vi "运维调试_采配水.vi"() -> ()   [LabVIEW 2016, in "PLC.lvlib"]
uses:
  PLC.lvlib
  <vilib>/Plasmionique/MB Master/MB_Master/MB_Master.lvclass
  <vilib>/Utility/miscctls.llb/LVPointTypeDef.ctl
  <vilib>/Plasmionique/MB Master/MB_Master_Serial/MB_Master_Serial.lvclass
  C:/Program Files (x86)/National Instruments/LabVIEW 2016/vi.lib/Plasmionique/MB Master/MB_Master/MB_Master.lvclass
  <vilib>/Instr/_visa.llb/VISA Configure Serial Port (Instr).vi
  <vilib>/NI/Modbus Library/API/Wrapper/Create TCP Slave.vi
  <vilib>/NI/Modbus Library/API/Slave/Modbus Slave.lvclass
  <vilib>/Plasmionique/MB Master/MB Master.lvlib
  <vilib>/NI/Modbus Library/API/Wrapper/API Main.lvlib
panel:
  out "Registers":u16[](array[numeric])
  out "R118":i16 caption="多参数沉淀时间"
  in  "看门狗启用":bool
  out "R117":i16 caption="看门狗设置值"
  out "R33":i16 caption="看门狗计时器"
  in  "下载模式":bool
  in  "R116":i16(ring) caption="储水水体选择" items=["自来水", "采水泵"]
  out "当前启动泵号":u16(ring) items=["1号水样泵", "2号水样泵"]
  out "R113":i16 caption="储水时间设定"
  out "R25":i16
  in  "V14NC":bool
  out "R24":i16
  in  "V14NO":bool
  out "X2":bool caption="X1"
  out "采配水版本号":string
  out "R23":i16 caption="清洗频次计数"
  out "R112":i16 caption="清洗频次设定"
  out "R22":i16
  in  "V13NC":bool
  out "R111":i16 caption="排液时间"
  out "通讯故障":bool
  out "R21":i16
  in  "V13NO":bool
  out "R20":i16
  in  "M1-2":bool
  in  "潜水泵工作模式":u16(ring) items=["泵1单泵单管路", "泵2单泵单管路", "潜水泵双泵双管路", "自吸泵双泵双管路"]
  out "X11":bool caption="废液报警"
  out "X10":bool caption="自来水检测"
  out "X9":bool caption="泵2过载报警"
  out "X8":bool caption="泵1过载报警"
  out "X7":bool caption="断电检测"
  out "X6":bool caption="开门检测"
  out "X5":bool caption="烟雾检测"
  out "X4":bool caption="漏水检测"
  out "X3":bool caption="进样检测"
  out "X1":bool
  out "X0":bool caption="采样池液位开关"
  out "R109":i16 caption="配水时间"
  out "集成报警信息":string
  out "R108":i16 caption="自来水报警"
  out "R107":i16 caption="采水池液位报警设置"
  out "R106":i16 caption="进样超时设置"
  out "R105":i16 caption="二级清洗时间"
  out "R104":i16 caption="一级清洗时间"
  out "R103":i16 caption="外部管路清洗时间"
  out "R102":i16 caption="静置沉淀时间"
  out "R101":i16 caption="内部管路润洗时间"
  out "R100":i16 caption="外部管路润洗时间"
  out "R2":i16
  out "R1":i16
  out "多列列表框":i32(listbox)
  out "R19":i16
  in  "V6":bool
  out "R18":i16
  in  "V5":bool
  out "R17":i16
  in  "V4":bool
  out "R16":i16
  in  "V3":bool
  out "R15":i16
  in  "V2":bool
  out "R14":i16
  in  "M2":bool
  out "R13":i16
  in  "V1":bool
  out "R12":i16
  in  "M1-1":bool
  in  "返回":bool
  in  "参数设置":bool
  in  "单步启动":bool
  in  "启动":bool
  in  "停止":bool
  # "看门狗设置"
  # "S"
  # "S"
  # "S"
  # "S"
  # "次"
  # "次"
  # "S"
  # "S"
  # "S"
  # "S"
  # "S"
  # "S"
  # "S"
  # "S"
  # "S"
  # "S"
  # "S"
  # "单步计时："
  # "s"
  # "流程计时："
  # "s"
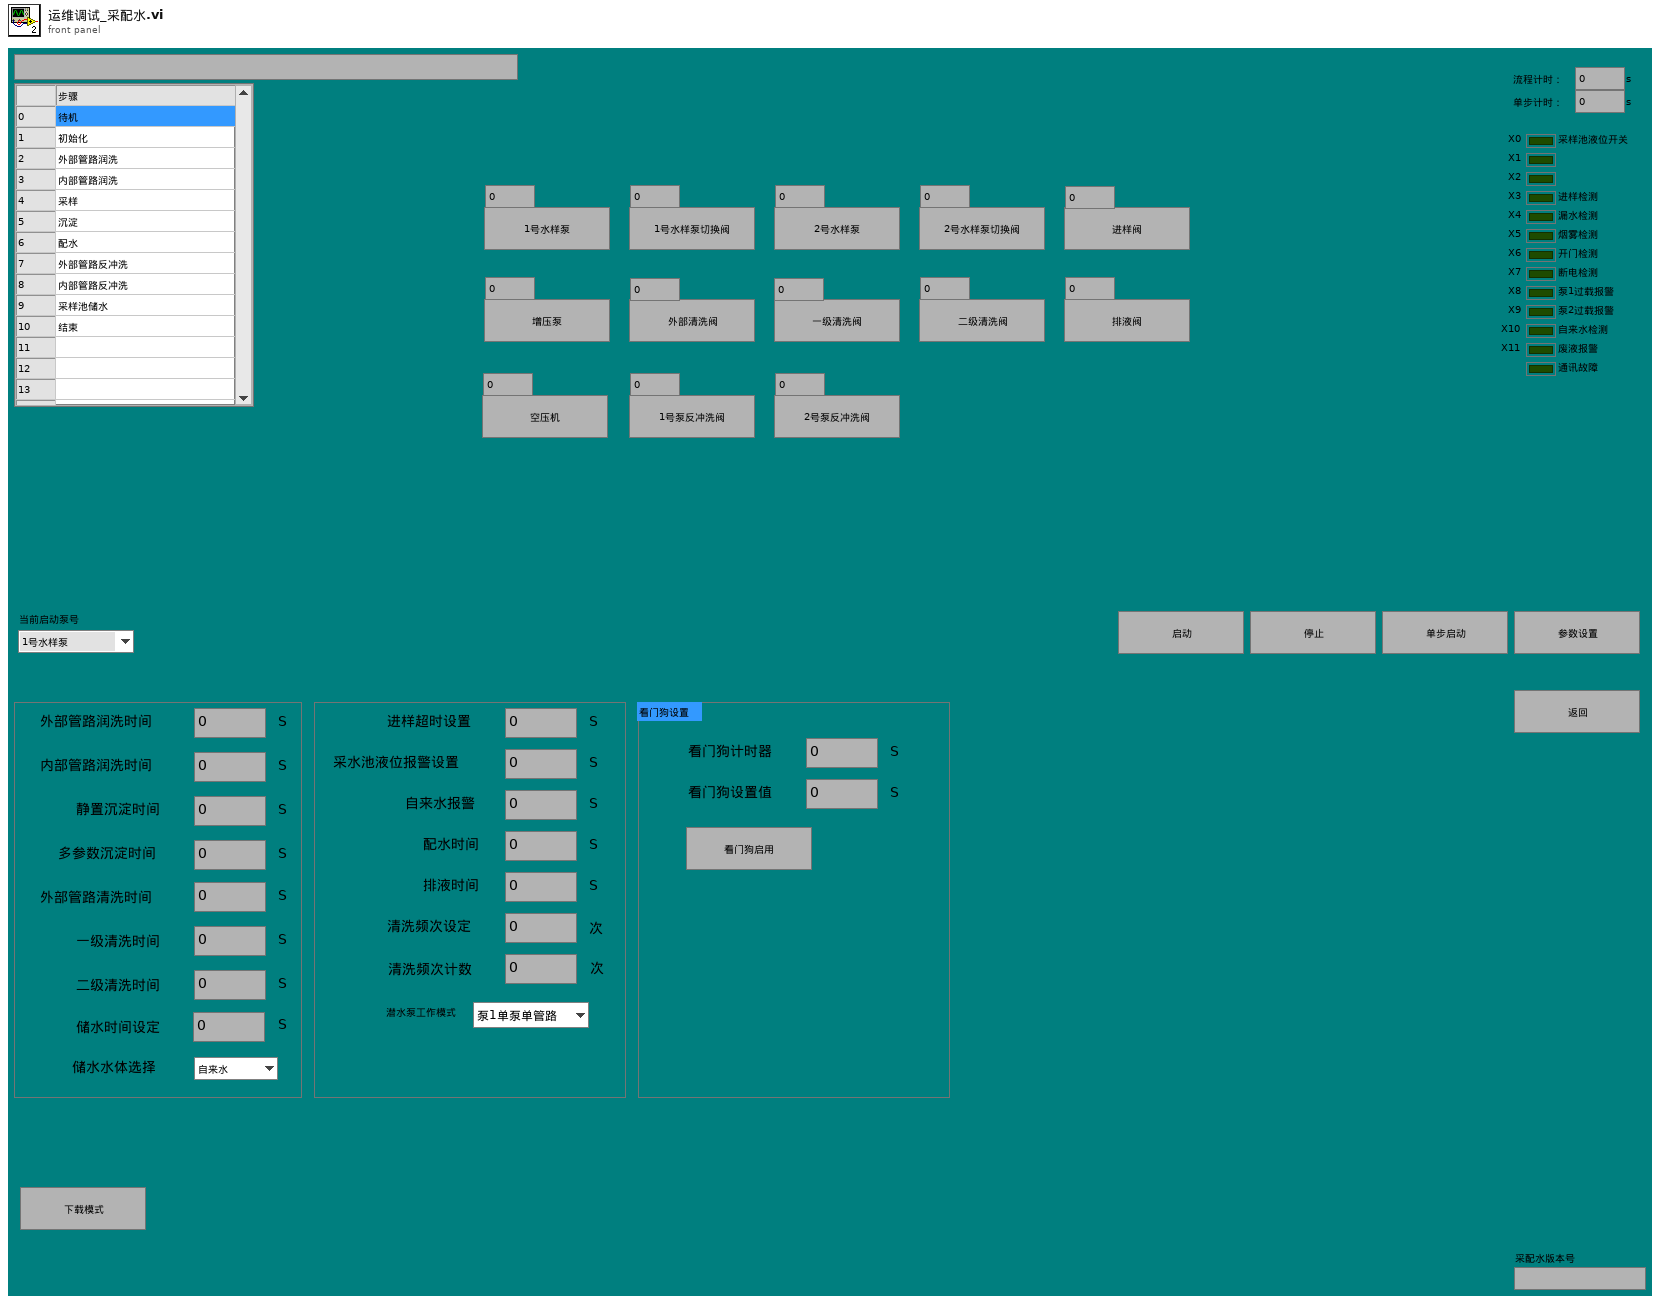
[diagram p1: front panel]
types:
  T1 = typedef "LVPointTypeDef.ctl" = cluster{"Horizontal":i16, "Vertical":i16}
  T2 = cluster{"命令":string, "数据":cluster{"starting address":u16, "holding register value":u16}}
  T3 = cluster{"时间标识":timestamp, "设备":string, "日志信息":string}
  T4 = cluster{"R0":i16, "R1":i16, "R2":i16, "R3":i16, "R4":i16, "R5":i16, "R6":i16, "R7":i16, "R8":i16, "R9":i16, "R10":i16, "R11":i16, "R12":i16, "R13":i16, "R14":i16, "R15":i16, "R16":i16, "R17":i16, "R18":i16, "R19":i16, "R20":i16, "R21":i16, "R22":i16, "R23":i16, "R24":i16, "R25":i16, "R26":i16, "R27":i16, "R28":i16, "R29":i16, "R30":i16, "R31":i16, "R32":i16, "R33":i16, "R34":i16}
  T5 = cluster{"R100":i16, "R101":i16, "R102":i16, "R103":i16, "R104":i16, "R105":i16, "R106":i16, "R107":i16, "R108":i16, "R109":i16, "R110":i16, "R111":i16, "R112":i16, "R113":i16, "R114":i16, "R115":i16, "R116":i16, "R117":i16, "R118":i16, "R119":i16}
  T6 = cluster{"seconds since 1Jan1904":timestamp, "table输入":string, string, "table输入":string}
  T7 = cluster{"时间标识":timestamp, "设备":string, "日志信息":string, "流程参数":string}
  T8 = cluster{"命令":string, cluster{"starting address":u16, "holding register value":u16}}
  T9 = cluster{"命令":string, "数据":cluster{"starting address":u16, "holding register values":u16[]}}
  T10 = cluster{"命令":string, "data":cluster{"starting address":u16, "coil values":bool[]}}
  T11 = cluster{"测试模式":enum16{"正常测试", "集成干预"}, "参数启用":cluster{"氨氮":bool, "总磷总氮":bool, "CODMn":bool, "CODcr":bool, "多参数":bool, "超标留样":bool}}
  T12 = enum32{"Bad", "Idle", "Run top level", "Running"}
  T13 = cluster{"baud rate (bps)":u32, "stop bits":u16, "parity":u16, "flow control":u16, "timeout":u32, "retries":i32}
  T14 = cluster{"starting address":u16, "holding register values":u16[]}
  T15 = cluster{"starting address":u16, "holding register value":u16}
  T16 = cluster{"starting address":u16, "coil values":bool[]}
  T17 = cluster{"Registers[0]":u16, "Registers[1]":u16, "Registers[2]":u16, "Registers[3]":u16, "Registers[4]":u16, "Registers[5]":u16, "Registers[6]":u16, "Registers[7]":u16, "Registers[8]":u16, "Registers[9]":u16, "Registers[10]":u16, "Registers[11]":u16, "Registers[12]":u16, "Registers[13]":u16, "Registers[14]":u16, "Registers[15]":u16, "Registers[16]":u16, "Registers[17]":u16, "Registers[18]":u16, "Registers[19]":u16, "Registers[20]":u16, "Registers[21]":u16, "Registers[22]":u16, "Registers[23]":u16, "Registers[24]":u16, "Registers[25]":u16, "Registers[26]":u16, "Registers[27]":u16, "Registers[28]":u16, "Registers[29]":u16, "Registers[30]":u16, "Registers[31]":u16, "Registers[32]":u16, "Registers[33]":u16, "Registers[34]":u16}
  T18 = cluster{"Registers[0]":u16, "Registers[1]":u16, "Registers[2]":u16, "Registers[3]":u16, "Registers[4]":u16, "Registers[5]":u16}
  T19 = cluster{"Registers[0]":u16, "Registers[1]":u16, "Registers[2]":u16, "Registers[3]":u16, "Registers[4]":u16, "Registers[5]":u16, "Registers[6]":u16, "Registers[7]":u16, "Registers[8]":u16, "Registers[9]":u16, "Registers[10]":u16, "Registers[11]":u16, "Registers[12]":u16, "Registers[13]":u16, "Registers[14]":u16, "Registers[15]":u16, "Registers[16]":u16, "Registers[17]":u16, "Registers[18]":u16, "Registers[19]":u16}
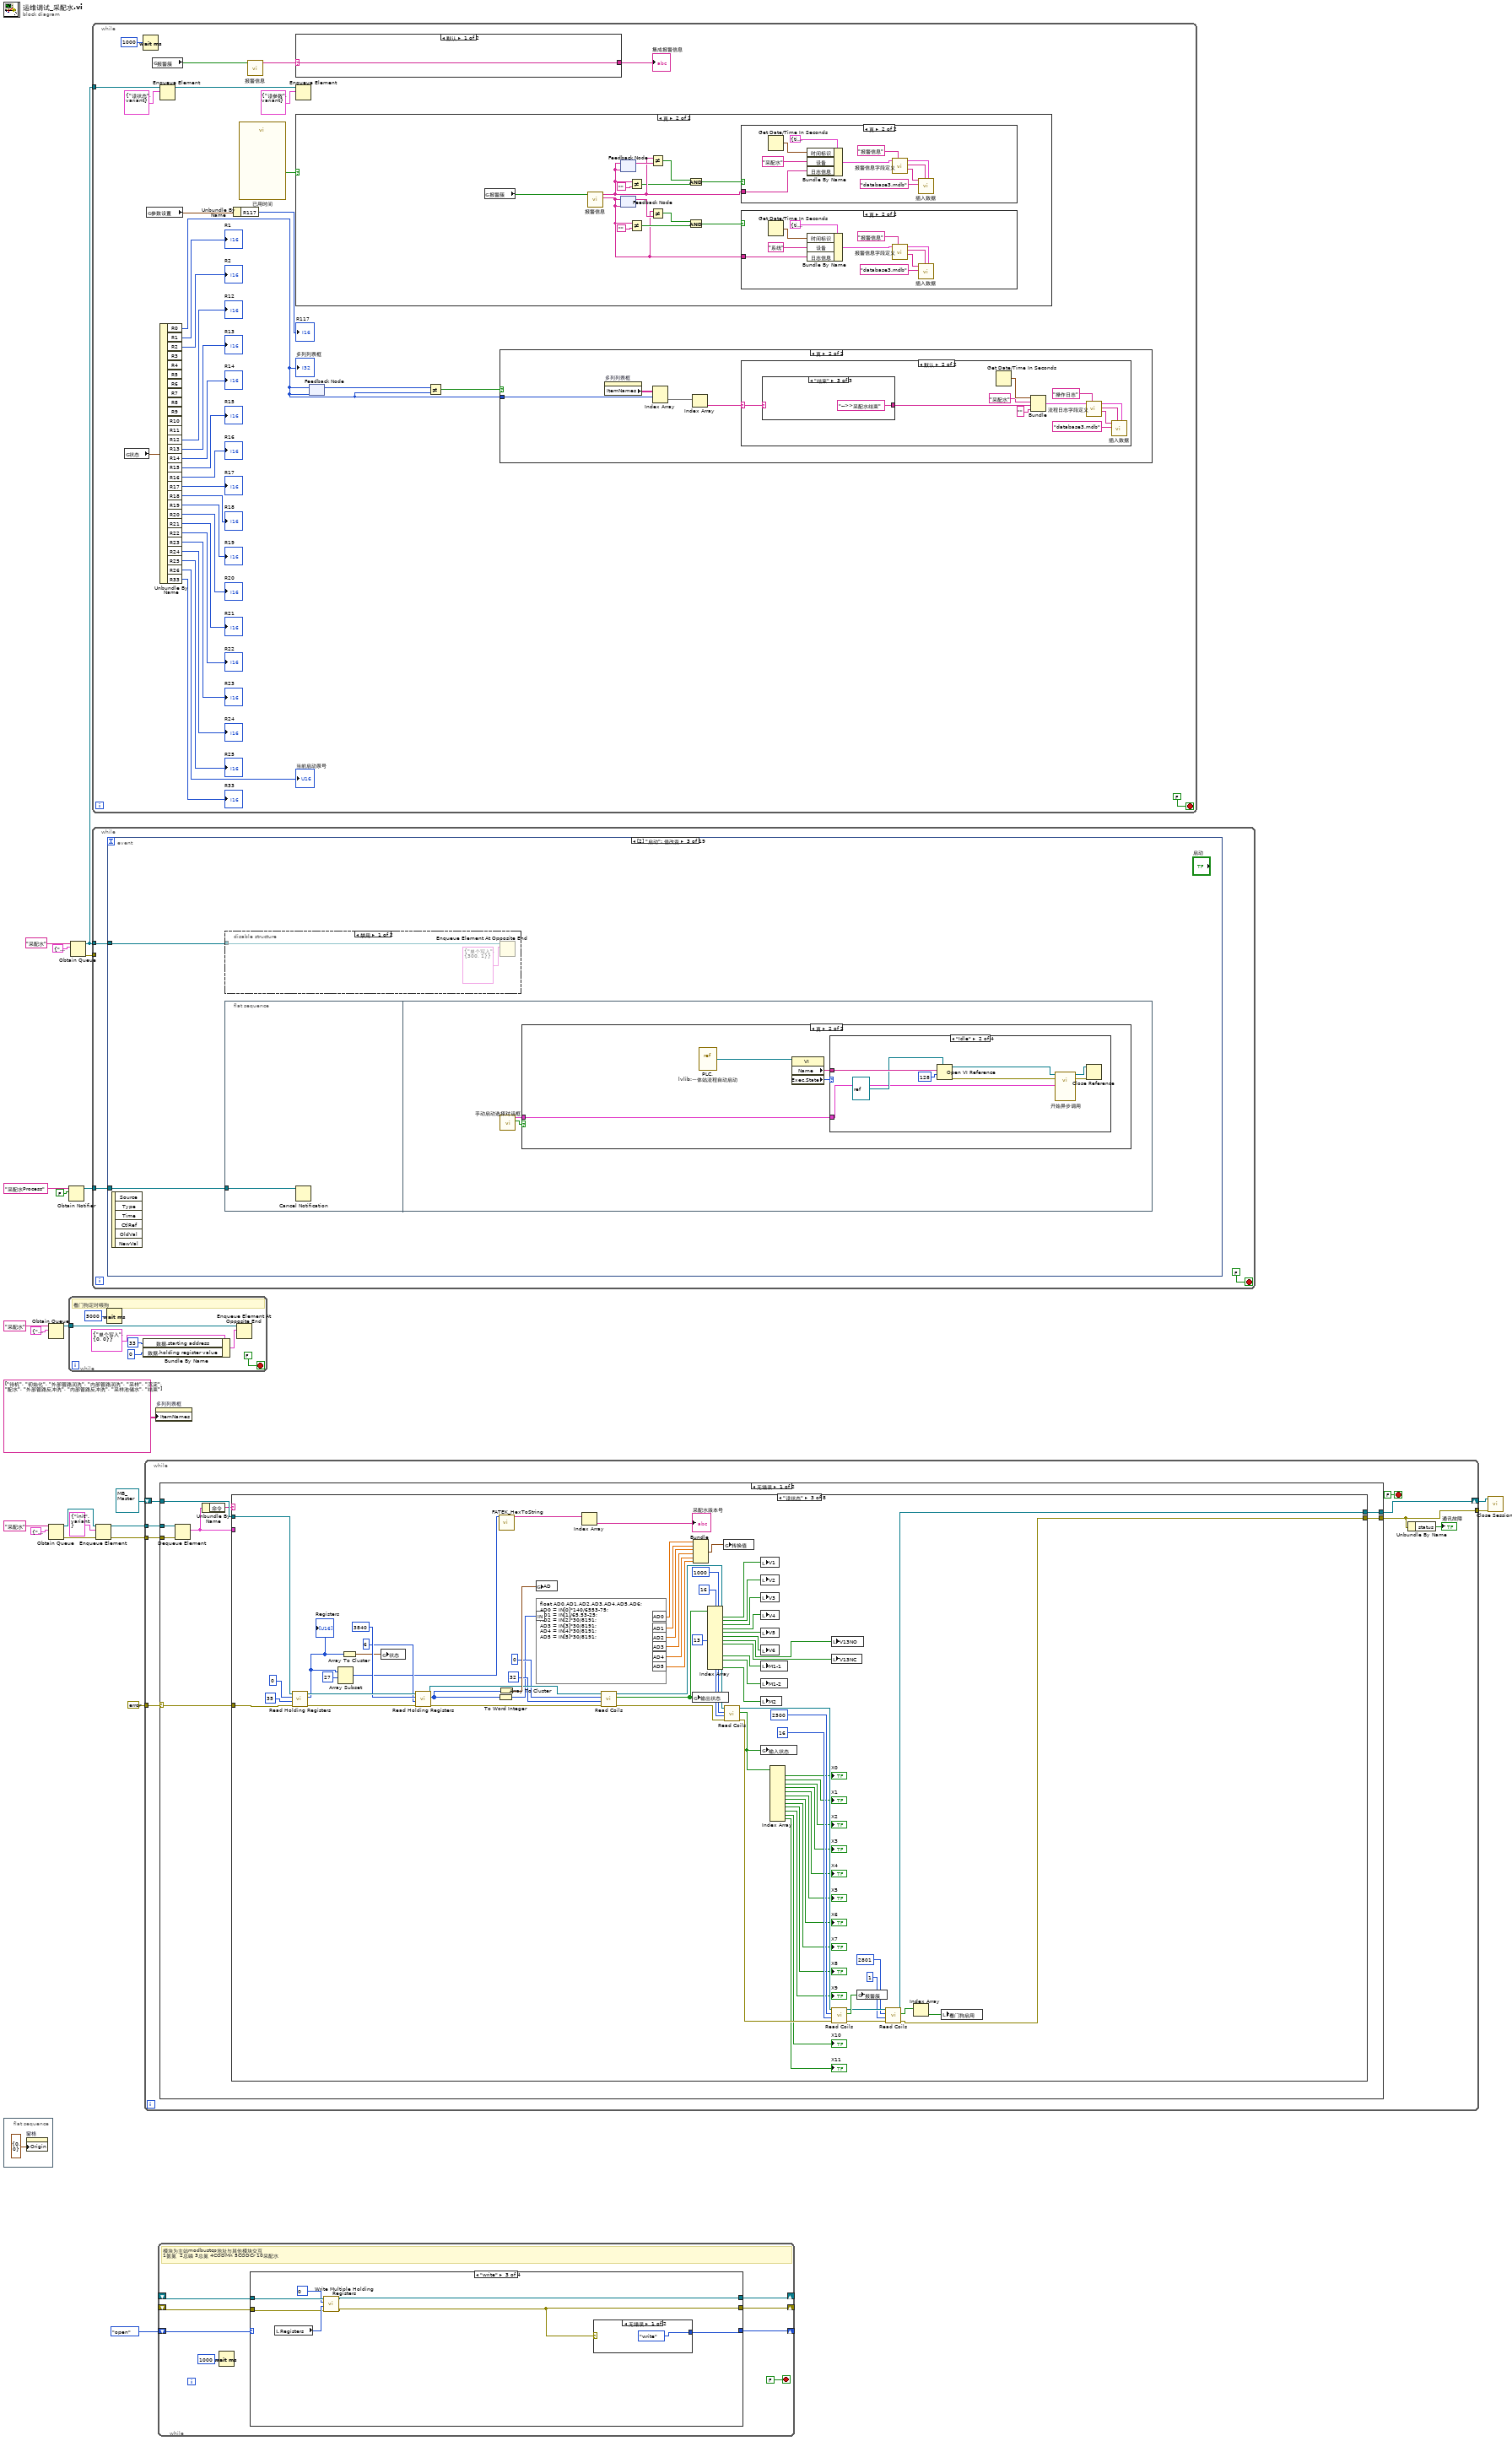
[diagram p0: block diagram]
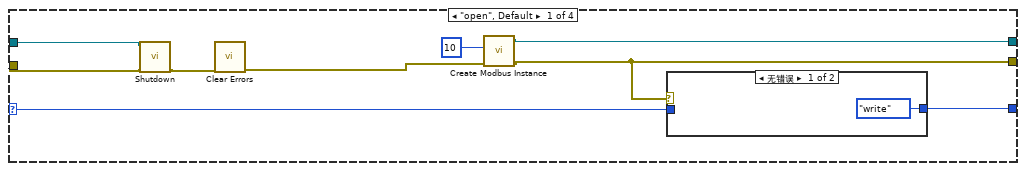
[diagram p2: hidden frame]
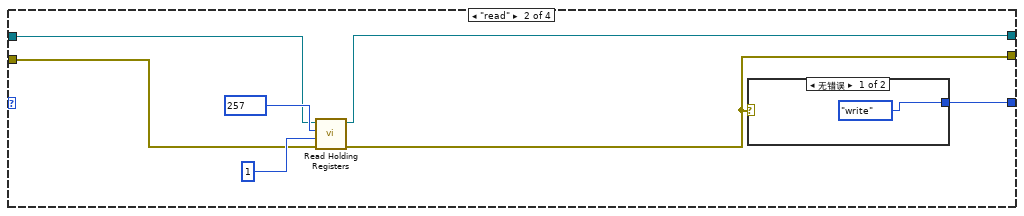
[diagram p4: hidden frame]
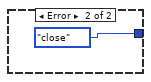
[diagram p5: hidden frame]
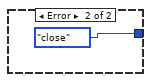
[diagram p6: hidden frame]
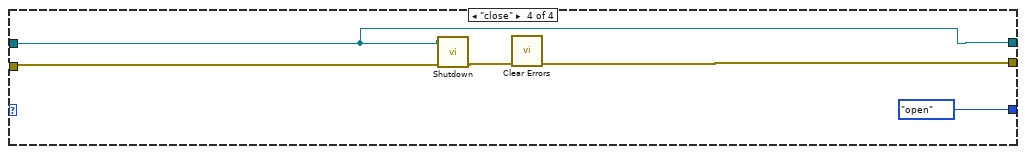
[diagram p7: hidden frame]
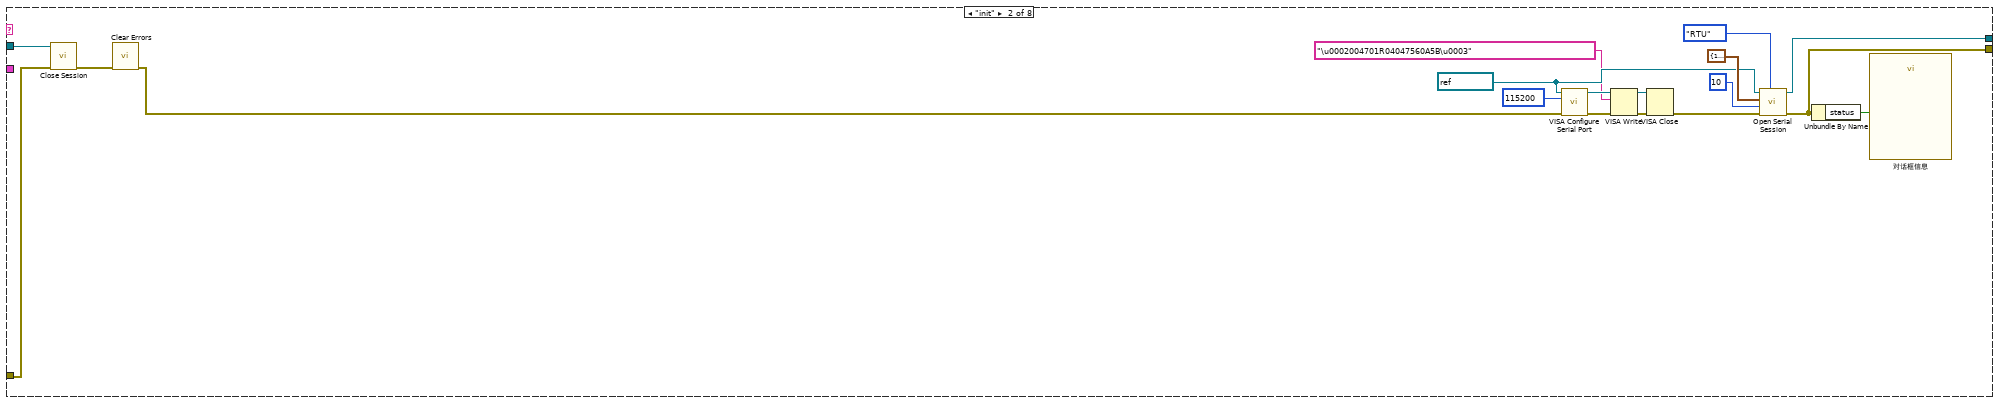
[diagram p9: hidden frame]
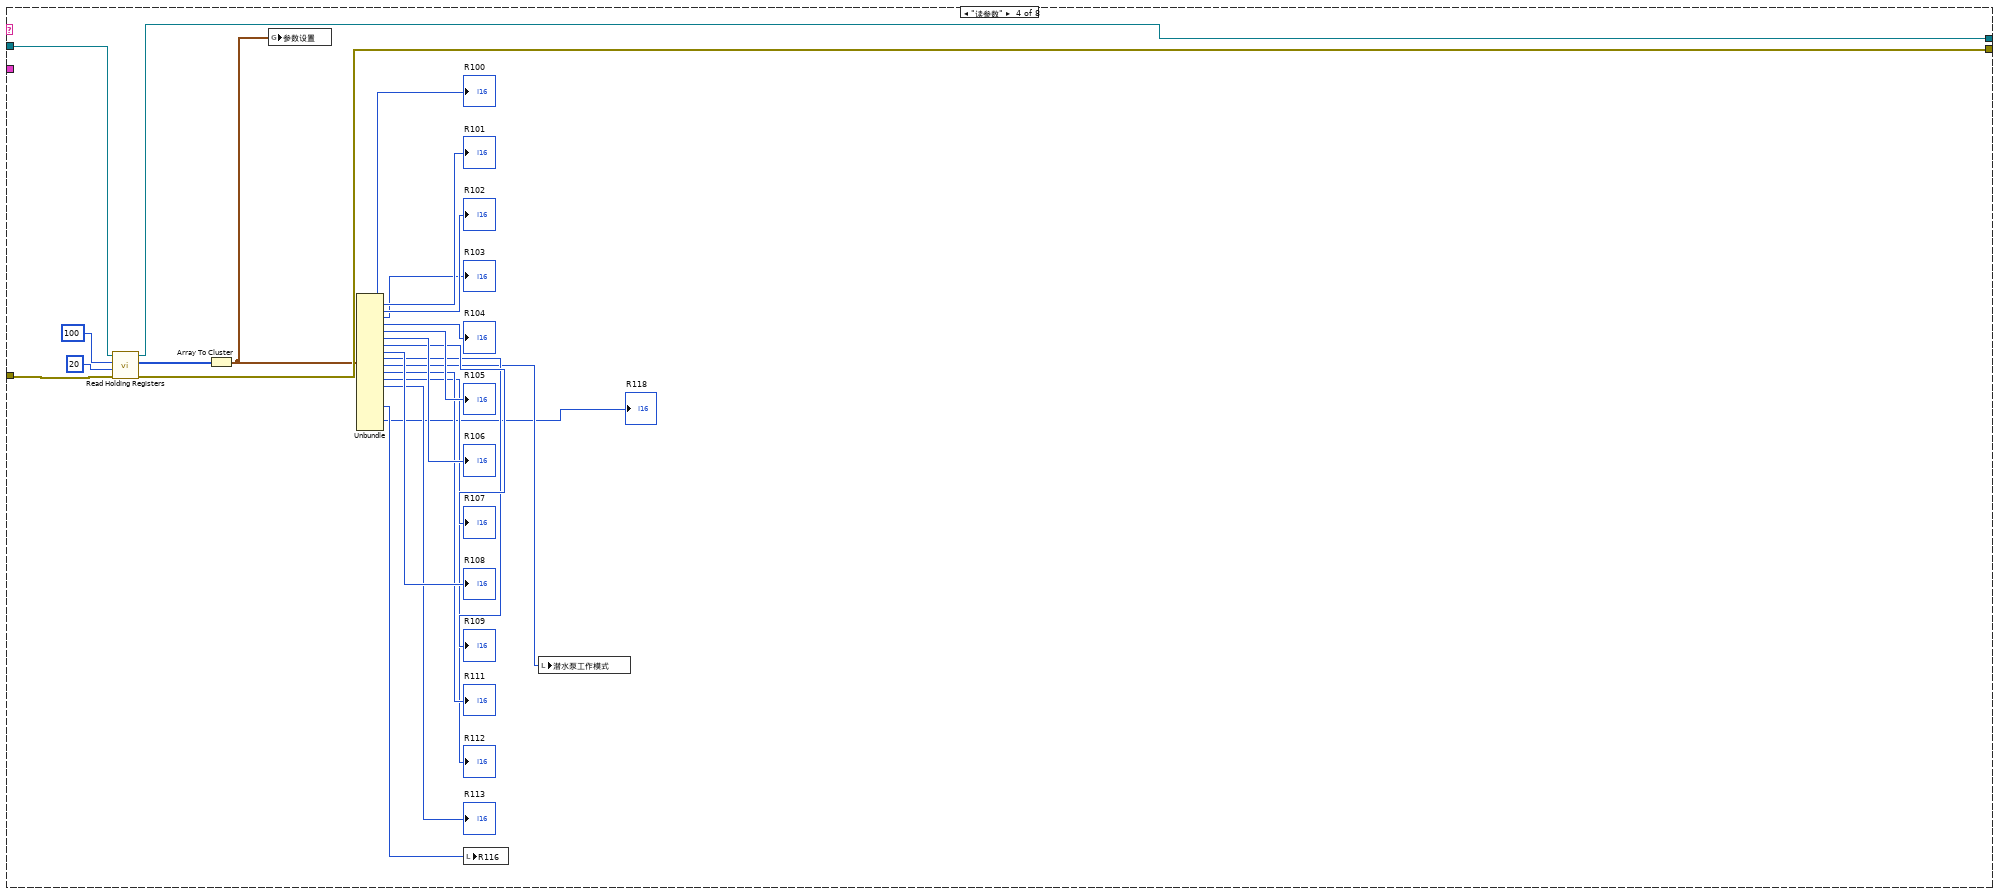
[diagram p10: hidden frame]
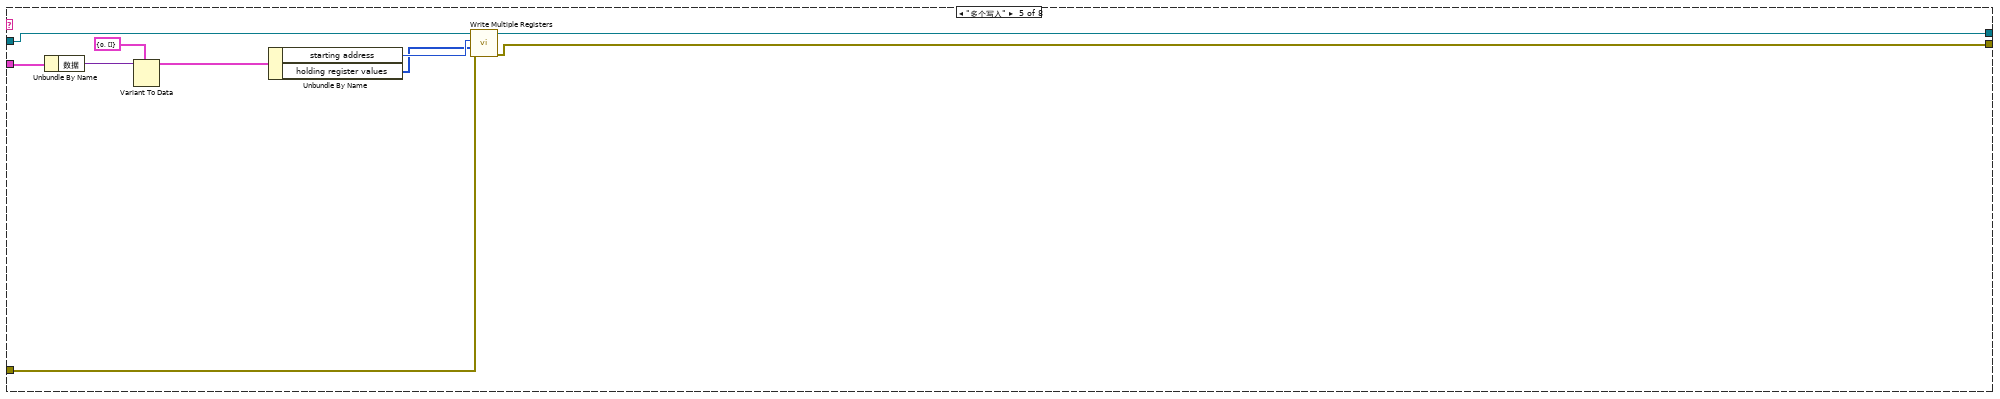
[diagram p11: hidden frame]
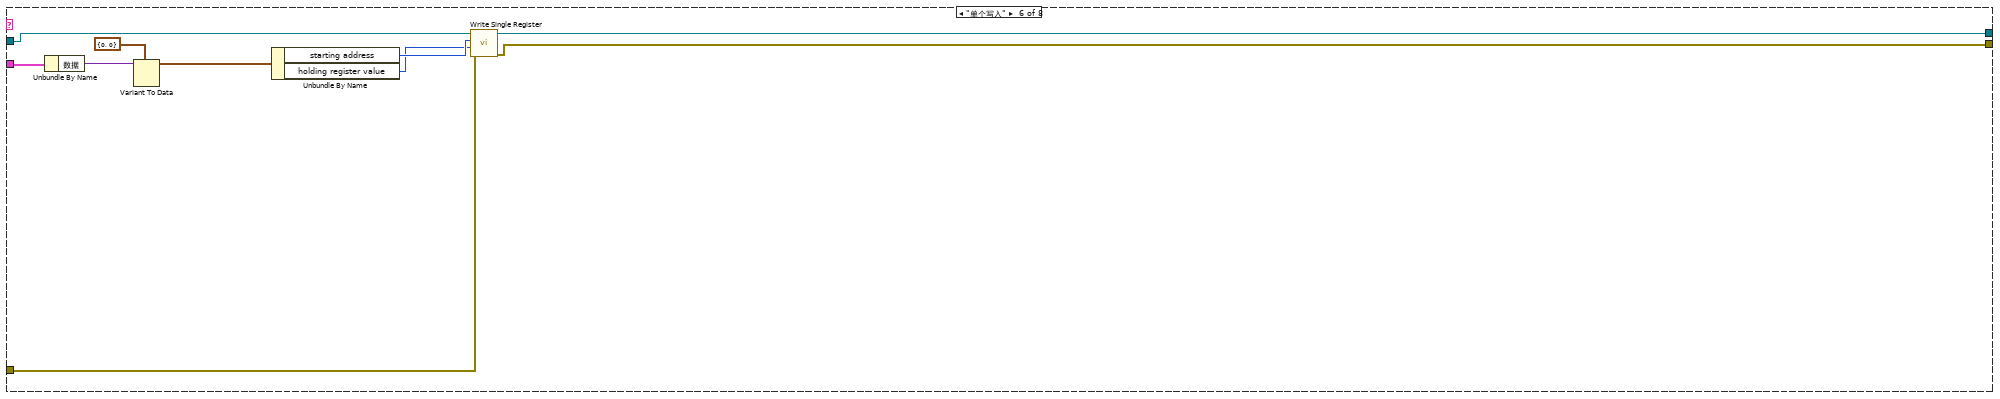
[diagram p12: hidden frame]
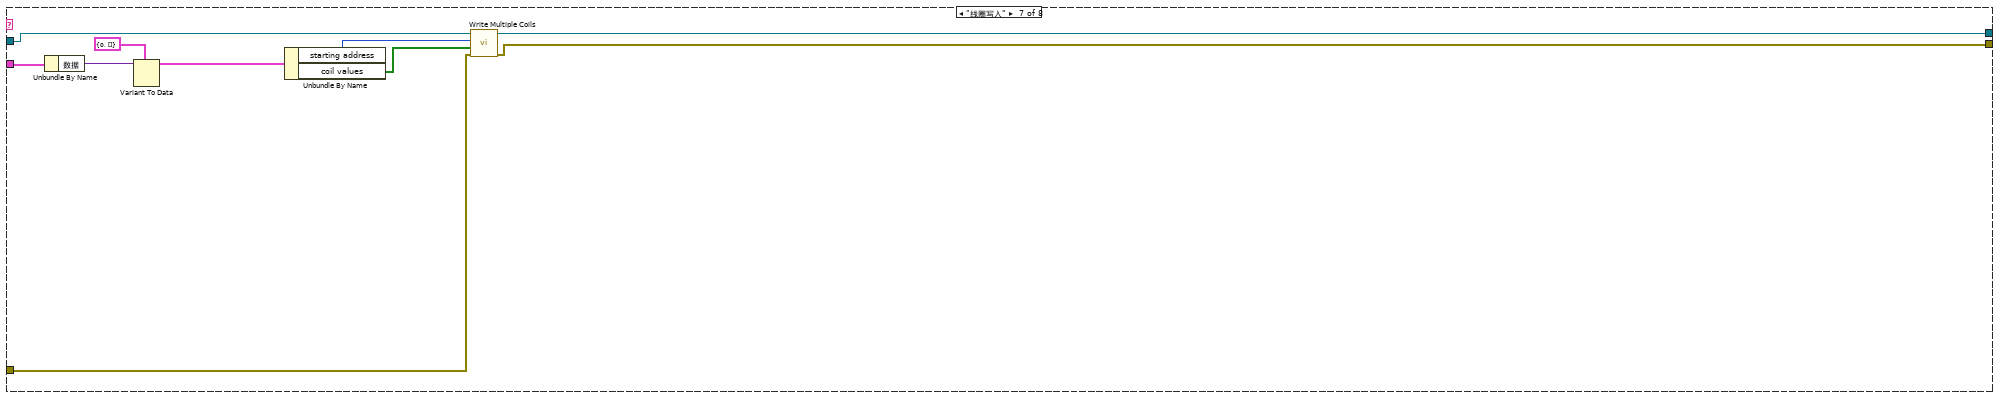
[diagram p13: hidden frame]
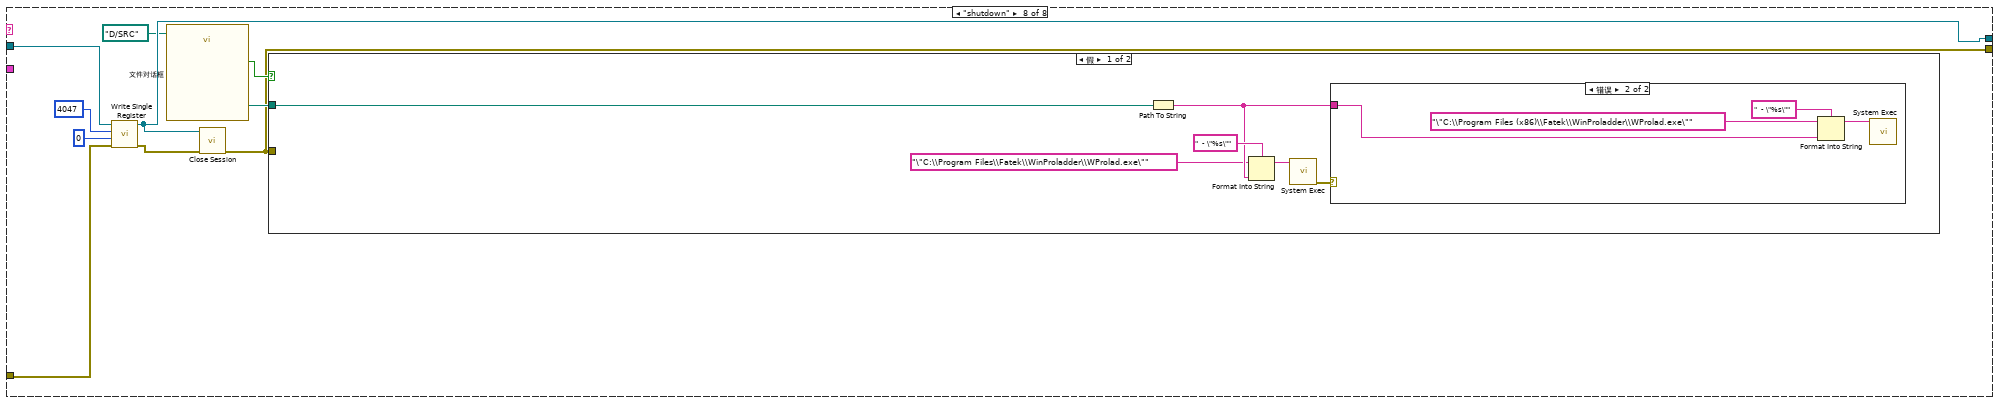
[diagram p14: hidden frame]
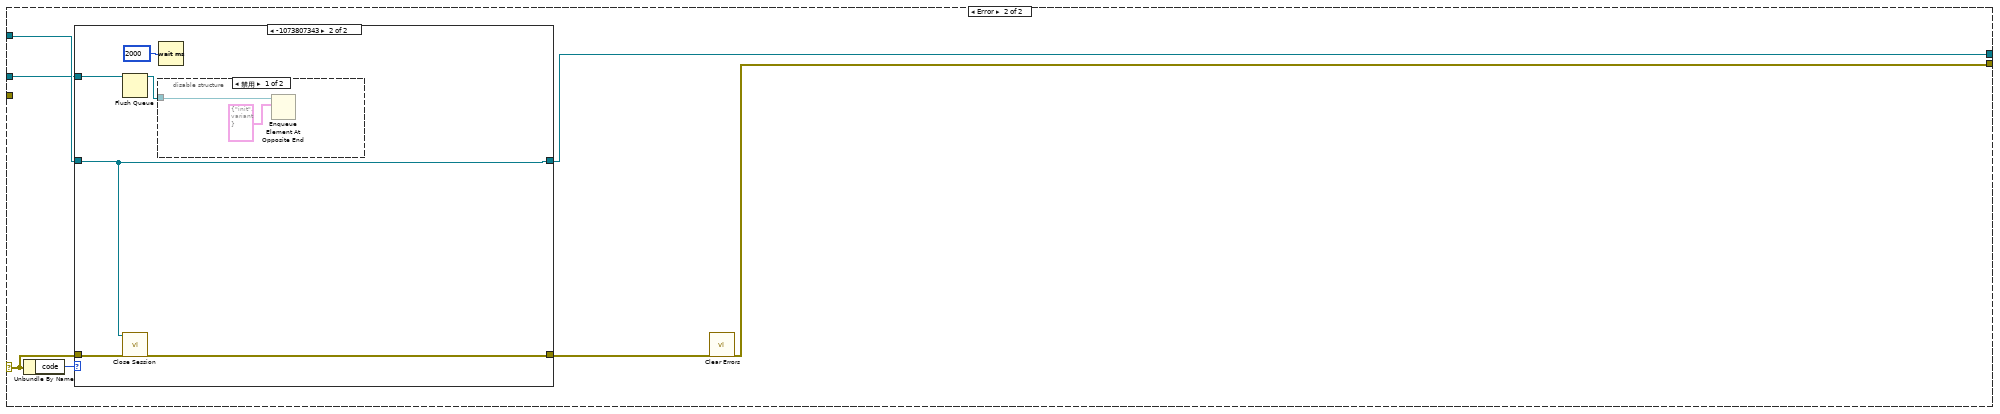
[diagram p17: hidden frame]
diagram:
  n1 = flat-sequence {
    frame #0 {
      n2 = property on="窗格" class="Pane"("Origin"=T1 {"Horizontal"=0, "Vertical"=0} ("原点")) -> ()  [unwired: 2 in, 2 out]
    }
  }
  n3 = Obtain Queue(name (unnamed)="采配水" ("名称（未命名）"), element data type=cluster{"命令":string, "数据":variant} {"命令"="", "数据"=variant}) -> (queue out=w2:refnum<queue>)  [unwired: 3 in, 2 out]
  n4 = Obtain Queue(name (unnamed)="采配水" ("名称（未命名）"), element data type=cluster{"命令":string, "数据":variant} {"命令"="", "数据"=variant}) -> (queue out=w13:refnum<queue>, error out=w12:errorcluster)  [unwired: 3 in, 1 out]
  n5 = Obtain Notifier(name (unnamed)="采配水Process" ("名称（未命名）"), notification data type=FALSE) -> (notifier out=w16:refnum<notifier>)  [unwired: 2 in, 2 out]
  n6 = while {
    tunnel: w2 -> [w27]
    stop <- FALSE stop-if-true
    # "看门狗定时喂狗"
    n7 = Wait (ms)(milliseconds to wait=u32 5000 ("等待时间（毫秒）")) -> ()  [unwired: 1 out]
    n8 = Bundle By Name(cluster=T2 {"命令"="单个写入", "数据"={"starting address"=0, "holding register value"=0}} ("元素"), "数据.starting address"=u16 33, "数据.holding register value"=u16 0) -> (w28:T2)
    n9 = Enqueue Element At Opposite End(queue=w27, element=w28) -> ()  [unwired: 2 in, 3 out]
  }
  n10 = Obtain Queue(name (unnamed)="采配水" ("名称（未命名）"), element data type=cluster{"命令":string, "数据":variant} {"命令"="", "数据"=variant}) -> (queue out=w20:refnum<queue>, error out=w21:errorcluster)  [unwired: 3 in, 1 out]
  n11 = while {
    tunnel: w20 -> [w64]
    stop <- FALSE stop-if-true
    n12 = global read "采配水全局变量.vi" "状态"() -> (w62:T4)
    n13 = Wait (ms)(milliseconds to wait=u32 1000 ("等待时间（毫秒）")) -> ()  [unwired: 1 out]
    n14 = global read "采配水全局变量.vi" "参数设置"() -> (w33:T5)
    n15 = global read "采配水全局变量.vi" "报警簇"() -> (w50:bool[])
    n16 = Enqueue Element(queue=w64, element=cluster{"命令":string, "数据":variant} {"命令"="读状态", "数据"=variant} ("元素")) -> (queue out=w45:refnum<queue>)  [unwired: 2 in, 2 out]
    n17 = Unbundle By Name(w62) -> ("R0"=w43:i16, "R1"=→"R1":i16, "R2"=→"R2":i16, "R12"=→"R12":i16, "R13"=→"R13":i16, "R14"=→"R14":i16, "R15"=→"R15":i16, "R16"=→"R16":i16, "R17"=→"R17":i16, "R18"=→"R18":i16, "R19"=→"R19":i16, "R20"=→"R20":i16, "R21"=→"R21":i16, "R22"=→"R22":i16, "R23"=→"R23":i16, "R24"=→"R24":i16, "R25"=→"R25":i16, "R26"=→"当前启动泵号":i16, "R33"=→"R33":i16)  [unwired: 9 out]
    "多列列表框" <- w43
    n18 = Unbundle By Name(w33) -> ("R117"=→"R117":i16)
    n19 = call "已用时间"() -> ("Time has Elapsed"=w48:bool)  [unwired: 12 in, 7 out]
    n20 = call "报警信息.vi"("报警簇"=w50) -> ("采配水报警信息"=w42:string)  [unwired: 9 in, 1 out]
    n21 = case shown="默认" w42 {
      selector: w42 -> [w99 _]
      tunnel: [w99 w100] -> w49
      frame Default {
      }
      frame "" {
        n22 = global read "采配水全局变量.vi" "运行状态显示"() -> (w100:string)
      }
    }
    "集成报警信息" <- w49
    n23 = Enqueue Element(queue=w45, element=cluster{"命令":string, "数据":variant} {"命令"="读参数", "数据"=variant} ("元素")) -> ()  [unwired: 2 in, 3 out]
    n24 = case shown="真" w48 {
      frame False {
      }
      frame True {
        n25 = global read "采配水全局变量.vi" "报警簇"() -> (w78:bool[])
        n26 = call "报警信息.vi"("报警簇"=w78) -> ("系统报警信息"=w67:string, "采配水报警信息"=w74:string)  [unwired: 9 in]
        n27 = feedback #1(w74) -> (w77:string)
        n28 = feedback-in #1(w74) -> ()
        n29 = feedback #2(w67) -> (w68:string)
        n30 = feedback-in #2(w67) -> ()
        n31 = Not Equal?(x=w74, y="") -> (x != y?=w72:bool)
        n32 = Not Equal?(x=w67, y="") -> (x != y?=w71:bool)
        n33 = Not Equal?(x=w74, y=w77) -> (x != y?=w76:bool)
        n34 = Not Equal?(x=w67, y=w68) -> (x != y?=w69:bool)
        n35 = And(x=w76, y=w72) -> (x .and. y?=w75:bool)
        n36 = And(x=w69, y=w71) -> (x .and. y?=w66:bool)
        n37 = case shown="真" w75 {
          tunnel: w74 -> [_ w89]
          frame False {
          }
          frame True {
            n38 = Get Date/Time In Seconds() -> (seconds since 1Jan1904=w91:timestamp)
            n39 = Bundle By Name(cluster=T3 {"时间标识"=timestamp(0 s since 1904-01-01), "设备"="", "日志信息"=""} ("data in"), "时间标识"=w91, "设备"="采配水", "日志信息"=w89) -> (w92:T3)
            n40 = call "报警信息字段定义.vi"("table输入"="报警信息", "data in"=w92) -> ("table输出"=w96:string, "columns"=w97:string[], "data out"=w98:T3)  [unwired: 7 in]
            n41 = call "插入数据.vi"("data"=w98, "columns"=w97, "database"="database3.mdb", "table"=w96) -> ()  [unwired: 7 in, 1 out]
          }
        }
        n42 = case shown="真" w66 {
          tunnel: w67 -> [_ w79]
          frame False {
          }
          frame True {
            n43 = Get Date/Time In Seconds() -> (seconds since 1Jan1904=w81:timestamp)
            n44 = Bundle By Name(cluster=T3 {"时间标识"=timestamp(0 s since 1904-01-01), "设备"="", "日志信息"=""} ("data in"), "时间标识"=w81, "设备"="系统", "日志信息"=w79) -> (w82:T3)
            n45 = call "报警信息字段定义.vi"("table输入"="报警信息", "data in"=w82) -> ("table输出"=w86:string, "columns"=w87:string[], "data out"=w88:T3)  [unwired: 7 in]
            n46 = call "插入数据.vi"("data"=w88, "columns"=w87, "database"="database3.mdb", "table"=w86) -> ()  [unwired: 7 in, 1 out]
          }
        }
      }
    }
    n47 = feedback-in #3(w43) -> ()
    n48 = feedback #3(w43) -> (w44:i16)
    n49 = Not Equal?(x=w44, y=w43) -> (x != y?=w51:bool)
    n50 = case shown="真" w51 {
      tunnel: w43 -> [_ w103]
      frame False {
      }
      frame True {
        n51 = property on="多列列表框" class="MCListbox (严格)"() -> ("ItemNames"=w104:string[][])  [unwired: 2 in, 2 out]
        n52 = Index Array(array=w104, index (row)=w103) -> (element=w102:string[])  [unwired: 1 in]
        n53 = Index Array(array=w102) -> (element=w101:string)  [unwired: 1 in]
        n54 = case shown="默认" w101 {
          selector: w101 -> [_ w106]
          frame "待机" {
          }
          frame Default {
            n55 = case shown="\"结束\"" w106 {
              selector: w106 -> [w116 _ _]
              tunnel: [w116 "-->>采配水初始化" "-->>采配水结束"] -> w105
              frame Default {
              }
              frame "初始化" {
              }
              frame "结束" {
              }
            }
            n56 = Get Date/Time In Seconds() -> (seconds since 1Jan1904=w110:timestamp)
            n57 = Bundle("seconds since 1Jan1904"=w110, "table输入"="采配水", w105, "table输入"="") -> (w108:T6)  [unwired: 1 in]
            n58 = call "流程日志字段定义.vi"("table输入"="操作日志", "data in"=w108) -> ("table输出"=w113:string, "columns"=w114:string[], "data out"=w115:T7)  [unwired: 7 in]
            n59 = call "插入数据.vi"("data"=w115, "columns"=w114, "database"="database3.mdb", "table"=w113) -> ()  [unwired: 7 in, 1 out]
          }
        }
      }
    }
  }
  n60 = while {
    tunnel: w20 -> [w120]
    tunnel: w21 -> [_]
    tunnel: w16 -> [w119]
    stop <- FALSE stop-if-true
    n61 = event shown="[2] \"启动\": 值改变" {
      selector: _ -> [_ _ _ _ _ _ _ _ _ _ _ _ _ _ _ _ _ _ _]
      dyn-events: _ -> [_ _ _ _ _ _ _ _ _ _ _ _ _ _ _ _ _ _ _]
      timeout: _ -> [_ _ _ _ _ _ _ _ _ _ _ _ _ _ _ _ _ _ _]
      tunnel: w120 -> [_ w124 w127 w149 w168 w173 w179 w190 _ _ _ _ w218 w220 w225 w230 w235 w240 w245]
      tunnel: w119 -> [_ w123 w126 _ _ _ _ _ _ _ _ _ _ _ _ _ _ _ _]
      event Timeout {
        n62 = event-data() -> ()  [unwired: 1 in, 3 out]
      }
      event "停止": Value Change {
        n63 = event-data() -> ()  [unwired: 1 in, 6 out]
        n64 = Send Notification(notification=TRUE ("通知"), notifier=w123) -> ()  [unwired: 1 in, 2 out]
        n65 = Enqueue Element At Opposite End(queue=w124, element=T8 {"命令"="单个写入", {"starting address"=300, "holding register value"=2}} ("元素")) -> ()  [unwired: 2 in, 3 out]
      }
      event "启动": Value Change {
        n66 = event-data() -> ()  [unwired: 1 in, 6 out]
        n67 = disable-structure shown="禁用" {
          disable-tunnel: w127 -> [w145 _]
          frame Disabled {
            n68 = Enqueue Element At Opposite End(queue=w145, element=T8 {"命令"="单个写入", {"starting address"=300, "holding register value"=1}} ("元素")) -> ()  [unwired: 2 in, 3 out]
          }
          frame Enabled {
          }
        }
        n69 = flat-sequence {
          tunnel: w126 -> [w128]
          frame #0 {
            n70 = Cancel Notification(0:w128) -> ()  [unwired: 1 in, 3 out]
          }
          frame #1 {
            n71 = call "手动启动选择对话框.vi"() -> ("确定"=w130:bool, "参数"=w129:T11)  [unwired: 10 in]
            n72 = case shown="真" w130 {
              tunnel: w129 -> [_ w131]
              frame False {
              }
              frame True {
                n73 = vi-ref "PLC.lvlib:一体站流程自动启动.vi"() -> (w134:refnum<vi>)
                n74 = property class="VI"(reference=w134) -> ("Name"=w133:string, "Exec.State"=w132:T12)  [unwired: 1 in, 2 out]
                n75 = case shown="\"Idle\"" w132 {
                  tunnel: w133 -> [_ w142 _ _]
                  tunnel: w131 -> [_ w135 _ _]
                  frame "Bad", Default {
                  }
                  frame "Idle" {
                    n76 = Open VI Reference(type specifier VI Refnum (for type only)=refnum<vi> refnum, vi path=w142, options=128 ("选项")) -> (vi reference=w140:refnum<vi>, error out=w138:errorcluster)  [unwired: 3 in]
                    n77 = call-by-ref "开始异步调用"(reference=w140, error in=w138, "参数"=w135) -> (reference out=w139:refnum<vi>, error out=w137:errorcluster)  [unwired: 11 in]
                    n78 = Close Reference(reference=w139, error in (no error)=w137) -> ()  [unwired: 1 out]
                  }
                  frame "Run top level" {
                  }
                  frame "Running" {
                    n79 = One Button Dialog(message="流程已经运行,无须重复启动" ("消息")) -> ()  [unwired: 1 in, 1 out]
                  }
                }
              }
            }
          }
        }
      }
      event "单步启动": Value Change {
        n80 = event-data() -> ()  [unwired: 1 in, 6 out]
        n81 = call "单步启动对话框.vi"() -> ("单步启动步骤输出"=w146:u16)  [unwired: 11 in]
        n82 = Bundle By Name(cluster=T2 {"命令"="单个写入", "数据"={"starting address"=301, "holding register value"=0}} ("元素"), "数据.holding register value"=w146) -> (w147:T2)
        n83 = Enqueue Element At Opposite End(queue=w149, element=w147) -> ()  [unwired: 2 in, 3 out]
      }
      event "R100", "R101", "R102", "R103", "R104", "R105", "R106", "R107", "R108", "R109", "潜水泵工作模式", "R111", "R112", "R113": Value Change {
        n84 = event-data() -> ()  [unwired: 1 in, 6 out]
        n85 = local read "R100"() -> (w163:i16)
        n86 = local read "R101"() -> (w162:i16)
        n87 = local read "R102"() -> (w161:i16)
        n88 = local read "R103"() -> (w160:i16)
        n89 = local read "R104"() -> (w159:i16)
        n90 = local read "R105"() -> (w158:i16)
        n91 = local read "R106"() -> (w157:i16)
        n92 = local read "R107"() -> (w156:i16)
        n93 = local read "R108"() -> (w155:i16)
        n94 = local read "R109"() -> (w154:i16)
        n95 = local read "R111"() -> (w152:i16)
        n96 = local read "R112"() -> (w151:i16)
        n97 = local read "R113"() -> (w150:i16)
        n98 = Build Array(w163, w162, w161, w160, w159, w158, w157, w156, w155, w154, "潜水泵工作模式", w152, w151, w150) -> (w164:u16[])
        n99 = Bundle By Name(cluster=T9 {"命令"="多个写入", "数据"={"starting address"=0, "holding register values"=[]}} ("元素"), "数据.starting address"=u16 100, "数据.holding register values"=w164) -> (w165:T9)
        n100 = Enqueue Element At Opposite End(queue=w168, element=w165) -> ()  [unwired: 2 in, 3 out]
      }
      event "R116", "R117", "R118": Value Change {
        n101 = event-data() -> ()  [unwired: 1 in, 6 out]
        n102 = local read "R117"() -> (w170:i16)
        n103 = local read "R118"() -> (w169:i16)
        n104 = Build Array("R116", w170, w169) -> (w172:i16[])
        n105 = Bundle By Name(cluster=T9 {"命令"="多个写入", "数据"={"starting address"=0, "holding register values"=[]}} ("元素"), "数据.starting address"=u16 116, "数据.holding register values"=w172) -> (w174:T9)
        n106 = Enqueue Element At Opposite End(queue=w173, element=w174) -> ()  [unwired: 2 in, 3 out]
      }
      event "下载模式": Value Change {
        n107 = event-data() -> ("NewVal"=w178:bool)  [unwired: 1 in, 5 out]
        n108 = Flush Queue(queue=w179) -> (queue out=w177:refnum<queue>)  [unwired: 1 in, 2 out]
        n109 = case shown="真" w178 {
          tunnel: w177 -> [w180 w184]
          frame False {
            n110 = Enqueue Element At Opposite End(queue=w180, element=cluster{"命令":string, "数据":variant} {"命令"="init", "数据"=variant} ("元素")) -> ()  [unwired: 2 in, 3 out]
          }
          frame True {
            n111 = Two Button Dialog(message="请再次确认是否切换为下载模式，切换为下载模式将导致采配水工作异常，非专业人员请勿进行此操作！" ("消息")) -> (T button?=w182:bool)  [unwired: 2 in]
            n112 = case shown="真" w182 {
              tunnel: w184 -> [_ w187]
              frame False {
                n113 = local write "下载模式"(FALSE ("下载模式")) -> ()
              }
              frame True {
                n114 = Enqueue Element At Opposite End(queue=w187, element=cluster{"命令":string, "数据":variant} {"命令"="shutdown", "数据"=variant} ("元素")) -> ()  [unwired: 2 in, 3 out]
              }
            }
          }
        }
      }
      event "R23": Value Change {
        n115 = event-data() -> ()  [unwired: 1 in, 6 out]
        n116 = local read "R23"() -> (w189:i16)
        n117 = Build Array(w189) -> (w188:i16[])
        n118 = Bundle By Name(cluster=T9 {"命令"="多个写入", "数据"={"starting address"=0, "holding register values"=[]}} ("元素"), "数据.starting address"=u16 23, "数据.holding register values"=w188) -> (w191:T9)
        n119 = Enqueue Element At Opposite End(queue=w190, element=w191) -> ()  [unwired: 2 in, 3 out]
      }
      event "R23": Mouse Down {
        n120 = event-data() -> ("CtlRef"=w196:refnum<vi>)  [unwired: 1 in, 7 out]
        n121 = Two Button Dialog(message="请确认是否更改，更改后将影响实际清洗频次" ("消息")) -> (T button?=w195:bool)  [unwired: 2 in]
        n122 = case shown="真" w195 {
          tunnel: w196 -> [_ w197]
          frame False {
          }
          frame True {
            n123 = property class="DigNum (严格)"(reference=w197) -> (reference out=w199:refnum<vi>, "Value"=w200:i16)  [unwired: 1 in, 1 out]
            n124 = call "数字键盘.vi"("OldNumber"=w200) -> ("NewNumber"=w198:sgl)
            n125 = property class="DigNum (严格)"(reference=w199, "Val(Sgnl)"=w198) -> ()  [unwired: 1 in, 2 out]
          }
        }
      }
      event "R100", "R101", "R102", "R103", "R104", "R105", "R106", "R107", "R108", "R109", "R111", "R112", "R113", "R117", "R118": Mouse Down {
        n126 = event-data() -> ("CtlRef"=w204:refnum<vi>)  [unwired: 1 in, 7 out]
        n127 = property class="DigNum (严格)"(reference=w204) -> (reference out=w202:refnum<vi>, "Value"=w203:i16)  [unwired: 1 in, 1 out]
        n128 = call "数字键盘.vi"("OldNumber"=w203) -> ("NewNumber"=w201:sgl)
        n129 = property class="DigNum (严格)"(reference=w202, "Val(Sgnl)"=w201) -> ()  [unwired: 1 in, 2 out]
      }
      event "参数设置": Value Change {
        n130 = event-data() -> ()  [unwired: 1 in, 6 out]
        n131 = property on="窗格" class="Pane"("Origin"=T1 {"Horizontal"=0, "Vertical"=628} ("原点")) -> ()  [unwired: 2 in, 2 out]
      }
      event "返回": Value Change {
        n132 = event-data() -> ()  [unwired: 1 in, 6 out]
        n133 = property on="窗格" class="Pane"("Origin"=T1 {"Horizontal"=0, "Vertical"=0} ("原点")) -> ()  [unwired: 2 in, 2 out]
      }
      event "M1-1", "V1", "M2", "V2", "V3", "V4", "V5", "V6": Value Change {
        n134 = event-data() -> ()  [unwired: 1 in, 6 out]
        n135 = Build Array("M1-1", "V1", "M2", "V2", "V3", "V4", "V5", "V6") -> (w207:bool[])
        n136 = Bundle By Name(cluster=T10 {"命令"="线圈写入", "data"={"starting address"=2400, "coil values"=[]}} ("元素"), "data.coil values"=w207) -> (w208:T10)
        n137 = Enqueue Element(queue=w218, element=w208) -> ()  [unwired: 2 in, 3 out]
      }
      event "M1-2": Value Change {
        n138 = event-data() -> ()  [unwired: 1 in, 6 out]
        n139 = Build Array("M1-2") -> (w221:bool[])
        n140 = Bundle By Name(cluster=T10 {"命令"="线圈写入", "data"={"starting address"=2413, "coil values"=[]}} ("元素"), "data.coil values"=w221) -> (w222:T10)
        n141 = Enqueue Element(queue=w220, element=w222) -> ()  [unwired: 2 in, 3 out]
      }
      event "看门狗启用": Value Change {
        n142 = event-data() -> ()  [unwired: 1 in, 6 out]
        n143 = Build Array("看门狗启用") -> (w226:bool[])
        n144 = Bundle By Name(cluster=T10 {"命令"="线圈写入", "data"={"starting address"=2801, "coil values"=[]}} ("元素"), "data.coil values"=w226) -> (w227:T10)
        n145 = Enqueue Element(queue=w225, element=w227) -> ()  [unwired: 2 in, 3 out]
      }
      event "V13NO": Value Change {
        n146 = event-data() -> ()  [unwired: 1 in, 6 out]
        n147 = Build Array("V13NO") -> (w231:bool[])
        n148 = Bundle By Name(cluster=T10 {"命令"="线圈写入", "data"={"starting address"=2414, "coil values"=[]}} ("元素"), "data.coil values"=w231) -> (w232:T10)
        n149 = Enqueue Element(queue=w230, element=w232) -> ()  [unwired: 2 in, 3 out]
      }
      event "V13NC": Value Change {
        n150 = event-data() -> ()  [unwired: 1 in, 6 out]
        n151 = Build Array("V13NC") -> (w236:bool[])
        n152 = Bundle By Name(cluster=T10 {"命令"="线圈写入", "data"={"starting address"=2415, "coil values"=[]}} ("元素"), "data.coil values"=w236) -> (w237:T10)
        n153 = Enqueue Element(queue=w235, element=w237) -> ()  [unwired: 2 in, 3 out]
      }
      event "V14NO": Value Change {
        n154 = event-data() -> ()  [unwired: 1 in, 6 out]
        n155 = Build Array("V14NO") -> (w241:bool[])
        n156 = Bundle By Name(cluster=T10 {"命令"="线圈写入", "data"={"starting address"=2408, "coil values"=[]}} ("元素"), "data.coil values"=w241) -> (w242:T10)
        n157 = Enqueue Element(queue=w240, element=w242) -> ()  [unwired: 2 in, 3 out]
      }
      event "V14NC": Value Change {
        n158 = event-data() -> ()  [unwired: 1 in, 6 out]
        n159 = Build Array("V14NC") -> (w246:bool[])
        n160 = Bundle By Name(cluster=T10 {"命令"="线圈写入", "data"={"starting address"=2409, "coil values"=[]}} ("元素"), "data.coil values"=w246) -> (w247:T10)
        n161 = Enqueue Element(queue=w245, element=w247) -> ()  [unwired: 2 in, 3 out]
      }
    }
  }
  n162 = Enqueue Element(queue=w13, element=cluster{"命令":string, "数据":variant} {"命令"="init", "数据"=variant} ("元素"), error in (no error)=w12) -> (queue out=w8:refnum<queue>, error out=w10:errorcluster)  [unwired: 1 in, 1 out]
  n163 = while {
    tunnel: w8 -> [w253]
    tunnel: w10 -> [w252]
    shift-right: [w256] -> w5
    shift-left: refnum<class "MB_Master.lvclass"> refnum ("MB session in") -> [w255]
    tunnel: errorcluster {"status"=FALSE, "code"=0, "source"=""} ("error out") -> [w254]
    tunnel: [w251] -> w6
    stop <- FALSE stop-if-true
    n164 = case shown="无错误" w254 {
      selector: w254 -> [w261 w434]
      tunnel: [w264 w433] -> w256
      tunnel: w255 -> [w263 w435]
      tunnel: [w262 w431] -> w251
      tunnel: w253 -> [w259 w430]
      tunnel: w252 -> [w258 _]
      frame No Error {
        n165 = Dequeue Element(queue=w259, error in (no error)=w258) -> (element=w257:cluster{"命令":string, "数据":variant})  [unwired: 1 in, 3 out]
        n166 = Unbundle By Name(w257) -> ("命令"=w260:string)
        n167 = case shown="\"读状态\"" w260 {
          tunnel: [w266 w279 w292 w374 w386 w396 w406 w416] -> w264
          tunnel: w263 -> [w266 w281 w344 w379 w389 w399 w409 w419]
          tunnel: [w265 w280 w290 w373 w387 w397 w407 w410] -> w262
          tunnel: w261 -> [w265 w283 w347 w378 w388 w398 w408 w417]
          tunnel: w257 -> [_ _ _ _ w385 w395 w405 _]
          frame "idle", Default {
          }
          frame "init" {
            w271 = refnum<visa-resource-name> "COM3" ("VISA resource name")
            n168 = call-dynamic "Close Session.vi"("error in (no error)"=w283, "MB session in"=w281) -> ("error out"=w282:errorcluster)  [unwired: 9 in]
            n169 = call <vilib>:"Clear Errors.vi"("error in (no error)"=w282) -> ("error out"=w269:errorcluster)  [unwired: 5 in, 1 out]
            n170 = call-poly "VISA Configure Serial Port"("VISA resource name"=w271, "baud rate (9600)"=u32 115200, "error in (no error)"=w269) -> ("VISA resource name out"=w273:refnum<visa-resource-name>, "error out"=w275:errorcluster)  [unwired: 11 in]
            n171 = VISA Write(VISA resource name=w273, write buffer="\u0002004701R04047560A5B\u0003" ("写入缓冲区"), error in (no error)=w275) -> (VISA resource name out=w272:refnum<visa-resource-name>, error out=w274:errorcluster)  [unwired: 1 out]
            n172 = VISA Close(VISA resource name=w272, error in (no error)=w274) -> (error out=w268:errorcluster)
            n173 = call <vilib>:"Open Serial Session.vi"("Mode (RTU)"=enum16{"RTU", "ASCII"}."RTU", "Error in"=w268, "Slave ID"=u8 10, "Serial Config"=T13 {"baud rate (bps)"=115200, "stop bits"=10, "parity"=0, "flow control"=0, "timeout"=500, "retries"=1}, "VISA Resource"=w271) -> ("Error out"=w280:errorcluster, "MB_Serial session"=w279:refnum<class "MB_Master_Serial.lvclass">)  [unwired: 5 in]
            n174 = Unbundle By Name(w280) -> ("status"=w284:bool)
            n175 = call "对话框信息"("Enable"=w284) -> ()  [unwired: 9 in, 2 out]
          }
          frame "读状态" {
            n176 = call <vilib>:"Read Holding Registers.vi"("error in (no error)"=w347, "quantity"=u16 35 ("number of holding registers"), "starting address"=u16 0, "MB session in"=w344) -> ("error out"=w342:errorcluster, "Registers"=w313:u16[], "MB session out"=w343:refnum<class "MB_Master.lvclass">)  [unwired: 5 in]
            "Registers" <- w313
            n177 = Array Subset(array=w313, index=27 ("索引")) -> (w311:u16[])  [unwired: 1 in]
            n178 = Array To Cluster(array=w313) -> (cluster=w285:T17)
            n179 = global write "采配水全局变量.vi" "状态"(w285) -> ()
            n180 = call <vilib>:"Read Holding Registers.vi"("error in (no error)"=w342, "quantity"=u16 6 ("number of holding registers"), "starting address"=u16 3840, "MB session in"=w343) -> ("error out"=w338:errorcluster, "Registers"=w315:u16[], "MB session out"=w339:refnum<class "MB_Master.lvclass">)  [unwired: 5 in]
            n181 = To Word Integer(number=w315) -> (16bit integer=w314:i16[])
            n182 = call "FATEK_HexToString.vi"("数组"=w311) -> ("STRING"=w310:string[])  [unwired: 10 in]
            n183 = Array To Cluster(array=w315) -> (cluster=w355:T18)
            n184 = global write "采配水全局变量.vi" "AD"(w355) -> ()
            n185 = formula code="float AD0,AD1,AD2,AD3,AD4,AD5,AD6;\nAD0 = IN[0]*140/6553-75;\nAD1 = IN[1]/65.53-25;\nAD2 = IN[2]*30/8191;\nAD3 = IN[3]*30/8191;\nAD4 = IN[4]*30/8191;\nAD5 = IN[5]*30/8191;"("IN"=w314) -> ("AD0"=w353:dbl, "AD1"=w352:dbl, "AD2"=w351:dbl, "AD3"=w350:dbl, "AD4"=w349:dbl, "AD5"=w348:dbl)
            n186 = Index Array(array=w310) -> (element=→"采配水版本号":string)  [unwired: 1 in]
            n187 = call <vilib>:"Read Coils.vi"("error in (no error)"=w338, "quantity"=u16 32 ("number of coils"), "starting address"=u16 0, "MB session in"=w339) -> ("error out"=w334:errorcluster, "Coils"=w319:bool[], "MB session out"=w335:refnum<class "MB_Master.lvclass">)  [unwired: 5 in]
            n188 = global write "采配水全局变量.vi" "输出状态"(w319) -> ()
            n189 = Bundle(w353, w352, w351, w350, w349, w348) -> (w354:cluster{dbl, dbl, dbl, dbl, dbl, dbl})  [unwired: 1 in]
            n190 = Index Array(array=w319, index #7=13 ("索引")) -> (element #1=w308:bool, element #2=w307:bool, element #3=w306:bool, element #4=w305:bool, element #5=w304:bool, element #6=w303:bool, element #7=w301:bool, element #8=w300:bool, element #11=w299:bool, element #12=w298:bool, element #14=w294:bool)  [unwired: 13 in, 3 out]
            n191 = global write "采配水全局变量.vi" "转换值"(w354) -> ()
            n192 = call <vilib>:"Read Coils.vi"("error in (no error)"=w334, "quantity"=u16 16 ("number of coils"), "starting address"=u16 1000, "MB session in"=w335) -> ("error out"=w330:errorcluster, "Coils"=w326:bool[], "MB session out"=w331:refnum<class "MB_Master.lvclass">)  [unwired: 5 in]
            n193 = local write "V1"(w308) -> ()
            n194 = local write "V2"(w307) -> ()
            n195 = local write "V3"(w306) -> ()
            n196 = local write "V4"(w305) -> ()
            n197 = local write "V5"(w304) -> ()
            n198 = local write "V6"(w303) -> ()
            n199 = local write "M1-1"(w299) -> ()
            n200 = local write "M1-2"(w298) -> ()
            n201 = local write "M2"(w294) -> ()
            n202 = global write "采配水全局变量.vi" "输入状态"(w326) -> ()
            n203 = Index Array(array=w326) -> (element #1=→"X0":bool, element #2=→"X1":bool, element #3=→"X2":bool, element #4=→"X3":bool, element #5=→"X4":bool, element #6=→"X5":bool, element #7=→"X6":bool, element #8=→"X7":bool, element #9=→"X8":bool, element #10=→"X9":bool, element #11=→"X10":bool, element #12=→"X11":bool)  [unwired: 12 in]
            n204 = local write "V13NO"(w301) -> ()
            n205 = local write "V13NC"(w300) -> ()
            n206 = call <vilib>:"Read Coils.vi"("error in (no error)"=w330, "quantity"=u16 16 ("number of coils"), "starting address"=u16 2500, "MB session in"=w331) -> ("error out"=w291:errorcluster, "Coils"=w327:bool[], "MB session out"=w293:refnum<class "MB_Master.lvclass">)  [unwired: 5 in]
            n207 = global write "采配水全局变量.vi" "报警簇"(w327) -> ()
            n208 = call <vilib>:"Read Coils.vi"("error in (no error)"=w291, "quantity"=u16 1 ("starting address"), "starting address"=u16 2801, "MB session in"=w293) -> ("error out"=w290:errorcluster, "Coils"=w287:bool[], "MB session out"=w292:refnum<class "MB_Master.lvclass">)  [unwired: 5 in]
            n209 = Index Array(array=w287) -> (element=w286:bool)  [unwired: 1 in]
            n210 = local write "看门狗启用"(w286) -> ()
          }
          frame "读参数" {
            n211 = call <vilib>:"Read Holding Registers.vi"("error in (no error)"=w378, "quantity"=u16 20 ("number of holding registers"), "starting address"=u16 100, "MB session in"=w379) -> ("error out"=w373:errorcluster, "Registers"=w375:u16[], "MB session out"=w374:refnum<class "MB_Master.lvclass">)  [unwired: 5 in]
            n212 = Array To Cluster(array=w375) -> (cluster=w362:T19)
            n213 = global write "采配水全局变量.vi" "参数设置"(w362) -> ()
            n214 = Unbundle(w362) -> ("Registers[0]"=→"R100":u16, "Registers[1]"=→"R101":u16, "Registers[2]"=→"R102":u16, "Registers[3]"=→"R103":u16, "Registers[4]"=→"R104":u16, "Registers[5]"=→"R105":u16, "Registers[6]"=→"R106":u16, "Registers[7]"=→"R107":u16, "Registers[8]"=→"R108":u16, "Registers[9]"=→"R109":u16, "Registers[10]"=w361:u16, "Registers[11]"=→"R111":u16, "Registers[12]"=→"R112":u16, "Registers[13]"=→"R113":u16, "Registers[16]"=w357:u16, "Registers[18]"=→"R118":u16)  [unwired: 4 out]
            n215 = local write "R116"(w357) -> ()
            n216 = local write "潜水泵工作模式"(w361) -> ()
          }
          frame "多个写入" {
            n217 = Unbundle By Name(w385) -> ("数据"=w384:variant)
            n218 = Variant To Data(type=T14 {"starting address"=0, "holding register values"=[]}, Variant=w384) -> (data=w382:T14)  [unwired: 1 in, 1 out]
            n219 = Unbundle By Name(w382) -> ("starting address"=w381:u16, "holding register values"=w380:u16[])
            n220 = call <vilib>:"Write Multiple Registers.vi"("error in (no error)"=w388, "values"=w380, "starting address"=w381, "MB session in"=w389) -> ("error out"=w387:errorcluster, "MB session out"=w386:refnum<class "MB_Master.lvclass">)  [unwired: 6 in]
          }
          frame "单个写入" {
            n221 = Unbundle By Name(w395) -> ("数据"=w394:variant)
            n222 = Variant To Data(type=T15 {"starting address"=0, "holding register value"=0}, Variant=w394) -> (data=w392:T15)  [unwired: 1 in, 1 out]
            n223 = Unbundle By Name(w392) -> ("starting address"=w391:u16, "holding register value"=w390:u16)
            n224 = call <vilib>:"Write Single Register.vi"("error in (no error)"=w398, "value"=w390, "address"=w391, "MB session in"=w399) -> ("error out"=w397:errorcluster, "MB session out"=w396:refnum<class "MB_Master.lvclass">)  [unwired: 6 in]
          }
          frame "线圈写入" {
            n225 = Unbundle By Name(w405) -> ("数据"=w404:variant)
            n226 = Variant To Data(type=T16 {"starting address"=0, "coil values"=[]}, Variant=w404) -> (data=w402:T16)  [unwired: 1 in, 1 out]
            n227 = Unbundle By Name(w402) -> ("starting address"=w401:u16, "coil values"=w400:bool[])
            n228 = call <vilib>:"Write Multiple Coils.vi"("error in (no error)"=w408, "values"=w400, "starting address"=w401, "MB session in"=w409) -> ("error out"=w407:errorcluster, "MB session out"=w406:refnum<class "MB_Master.lvclass">)  [unwired: 6 in]
          }
          frame "shutdown" {
            n229 = call <vilib>:"Write Single Register.vi"("error in (no error)"=w417, "value"=u16 0, "address"=u16 4047, "MB session in"=w419) -> ("error out"=w418:errorcluster, "MB session out"=w416:refnum<class "MB_Master.lvclass">)  [unwired: 6 in]
            n230 = call "文件对话框"("start path"=path "D:/SRC") -> ("selected path"=w413:path, "cancelled"=w411:bool)  [unwired: 11 in, 2 out]
            n231 = call-dynamic "Close Session.vi"("error in (no error)"=w418, "MB session in"=w416) -> ("error out"=w410:errorcluster)  [unwired: 9 in]
            n232 = case shown="假" w411 {
              tunnel: w413 -> [w424 _]
              tunnel: w410 -> [_ _]
              frame False {
                n233 = Path To String(path=w424) -> (string=w421:string)
                n234 = Format Into String(format string="  - \"%s\"" ("格式字符串"), initial string="\"C:\\Program Files\\Fatek\\WinProladder\\WProlad.exe\"" ("command line"), w421) -> (resulting string=w422:string)  [unwired: 1 in, 1 out]
                n235 = call <vilib>:"System Exec.vi"("command line"=w422) -> ("error out"=w425:errorcluster)  [unwired: 7 in, 3 out]
                n236 = case shown="错误" w425 {
                  tunnel: w421 -> [_ w428]
                  frame No Error {
                  }
                  frame Error {
                    n237 = Format Into String(format string="  - \"%s\"" ("格式字符串"), initial string="\"C:\\Program Files (x86)\\Fatek\\WinProladder\\WProlad.exe\"" ("command line"), w428) -> (resulting string=w426:string)  [unwired: 1 in, 1 out]
                    n238 = call <vilib>:"System Exec.vi"("command line"=w426) -> ()  [unwired: 7 in, 4 out]
                  }
                }
              }
              frame True {
              }
            }
          }
        }
      }
      frame Error {
        n239 = Unbundle By Name(w434) -> ("code"=w436:i32)
        n240 = case shown="-1073807343" w436 {
          tunnel: w435 -> [w438 w442]
          tunnel: w434 -> [w437 w444]
          tunnel: [w437 w443] -> w432
          tunnel: [w438 w442] -> w433
          tunnel: w430 -> [_ w441]
          frame Default {
          }
          frame -1073807343 {
            n241 = Flush Queue(queue=w441) -> (queue out=w440:refnum<queue>)  [unwired: 1 in, 2 out]
            n242 = call-dynamic "Close Session.vi"("error in (no error)"=w444, "MB session in"=w442) -> ("error out"=w443:errorcluster)  [unwired: 9 in]
            n243 = disable-structure shown="禁用" {
              disable-tunnel: w440 -> [w445 _]
              frame Disabled {
                n244 = Enqueue Element At Opposite End(queue=w445, element=cluster{"命令":string, "数据":variant} {"命令"="init", "数据"=variant} ("元素")) -> ()  [unwired: 2 in, 3 out]
              }
              frame Enabled {
              }
            }
            n245 = Wait (ms)(milliseconds to wait=u32 2000 ("等待时间（毫秒）")) -> ()  [unwired: 1 out]
          }
        }
        n246 = call <vilib>:"Clear Errors.vi"("error in (no error)"=w432) -> ("error out"=w431:errorcluster)  [unwired: 5 in, 1 out]
      }
    }
    n247 = Unbundle By Name(w251) -> ("status"=→"通讯故障":bool)
  }
  n248 = property on="多列列表框" class="MCListbox (严格)"("ItemNames"=string[][] [["待机"], ["初始化"], ["外部管路润洗"], ["内部管路润洗"], ["采样"], ["沉淀"], ["配水"], ["外部管路反冲洗"], ["内部管路反冲洗"], ["采样池储水"], ["结束"]] ("项名")) -> ()  [unwired: 2 in, 2 out]
  n249 = while {
    shift-right: [w452] -> _
    shift-left: _ -> [w454]
    shift-right: [w451] -> _
    shift-left: _ -> [w453]
    shift-right: [w448] -> _
    shift-left: enum16{"open", "read", "write", "close"}."open" -> [w449]
    stop <- FALSE stop-if-true
    # "模块为主站modbustcp地址与其他模块交互\n1氨氮  2总磷 3总氮 4CODMn 5CODCr 10采配水"
    n250 = Wait (ms)(milliseconds to wait=u32 1000 ("等待时间（毫秒）")) -> ()  [unwired: 1 out]
    n251 = case shown="\"write\"" w449 {
      selector: w449 -> [w463 _ _ _]
      tunnel: w454 -> [w457 w469 w480 w486]
      tunnel: w453 -> [w456 w468 w477 w485]
      tunnel: [w460 w466 w476 w486] -> w452
      tunnel: [w459 w467 w475 w488] -> w451
      tunnel: [w462 w472 w481 enum16{"open", "read", "write", "close"}."open"] -> w448
      frame "open", Default {
        n252 = call-dynamic "Shutdown.vi"("error in"=w456, "Modbus slave in"=w457) -> ("error out"=w455:errorcluster)  [unwired: 9 in]
        n253 = call <vilib>:"Clear Errors.vi"("error in (no error)"=w455) -> ("error out"=w458:errorcluster)  [unwired: 5 in, 1 out]
        n254 = call-poly <vilib>:"Create Modbus Instance.vi"("error in"=w458, "port (502)"=u16 10) -> ("error out"=w459:errorcluster, "TCP slave instance"=w460:refnum<class "Modbus Slave.lvclass">)  [unwired: 8 in]
        n255 = case shown="无错误" w459 {
          tunnel: w463 -> [_ w465]
          tunnel: [enum16{"open", "read", "write", "close"}."write" w465] -> w462
          frame No Error {
          }
          frame Error {
          }
        }
      }
      frame "read" {
        n256 = call-dynamic <vilib>:"Read Holding Registers.vi"("error in"=w468, "number of inputs"=u16 1, "starting address"=u16 257, "Modbus slave in"=w469) -> ("error out"=w467:errorcluster, "Modbus slave out"=w466:refnum<class "Modbus Slave.lvclass">)  [unwired: 5 in, 1 out]
        n257 = case shown="无错误" w467 {
          tunnel: [enum16{"open", "read", "write", "close"}."write" enum16{"open", "read", "write", "close"}."close"] -> w472
          frame No Error {
          }
          frame Error {
          }
        }
      }
      frame "write" {
        n258 = local read "Registers"() -> (w478:u16[])
        n259 = call-dynamic "Write Multiple Holding Registers.vi"("error in"=w477, "registers to write"=w478, "starting address"=u16 0, "Modbus slave in"=w480) -> ("error out"=w475:errorcluster, "Modbus slave out"=w476:refnum<class "Modbus Slave.lvclass">)  [unwired: 6 in]
        n260 = case shown="无错误" w475 {
          tunnel: [enum16{"open", "read", "write", "close"}."write" enum16{"open", "read", "write", "close"}."close"] -> w481
          frame No Error {
          }
          frame Error {
          }
        }
      }
      frame "close" {
        n261 = call-dynamic "Shutdown.vi"("error in"=w485, "Modbus slave in"=w486) -> ("error out"=w484:errorcluster)  [unwired: 9 in]
        n262 = call <vilib>:"Clear Errors.vi"("error in (no error)"=w484) -> ("error out"=w488:errorcluster)  [unwired: 5 in, 1 out]
      }
    }
  }
  n263 = call-dynamic "Close Session.vi"("error in (no error)"=w6, "MB session in"=w5) -> ()  [unwired: 9 in, 1 out]
